vi "Close Holes.vi"(9 "Start Angle":dbl, 11 "Preliminary Arc Size":dbl) -> (1 "Final Arc Size":dbl, 3 "Final Angle":dbl)   [LabVIEW 2016, in "CML UI.lvlib" / "Circular Cue Helper.lvlib"]
uses:
  Circular Cue Helper.lvlib
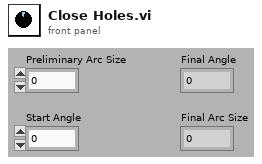
[diagram p1: front panel]
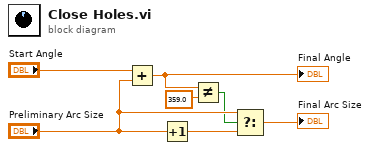
[diagram p0: block diagram]
diagram:
  n1 = Add(x="Start Angle", y="Preliminary Arc Size") -> (x+y=w5:dbl)
  "Final Angle" <- w5
  n2 = Increment(x="Preliminary Arc Size") -> (x+1=w6:dbl)
  n3 = Not Equal?(x=w5, y=359.0 ("x")) -> (x != y?=w3:bool)
  n4 = Select(t="Preliminary Arc Size", s=w3, f=w6) -> (s? t:f=→"Final Arc Size":dbl)
